vi "Found Four Edge.vi"(7 "Row ROI Name":string, 8 "error in":errorcluster, 9 "Calibration":T2, 10 "Template":T2, 11 "Image In":T2) -> (0 "error out":errorcluster, 1 "Array of Fitting":T1(array[cluster]), 2 "Match?":bool, 3 "Image out":T2, 4 "Elapsed time(ms)":u32)   [LabVIEW 2017]
uses:
  <vilib>/vision/Image Controls.llb/IMAQ Image.ctl
  Toolbox/Control/CVT Action.ctl
  <vilib>/vision/Measure.llb/Edge Options.ctl
  <vilib>/vision/Measure.llb/Edge Polarity.ctl
  <vilib>/vision/Measure.llb/Straight Edge Options.ctl
  <vilib>/vision/Measure.llb/Straight Edge Process.ctl
  Toolbox/Control/CVT name.vi
  Toolbox/Toolbox.lvlib
  <vilib>/vision/NI_Vision_Development_Module.lvlib
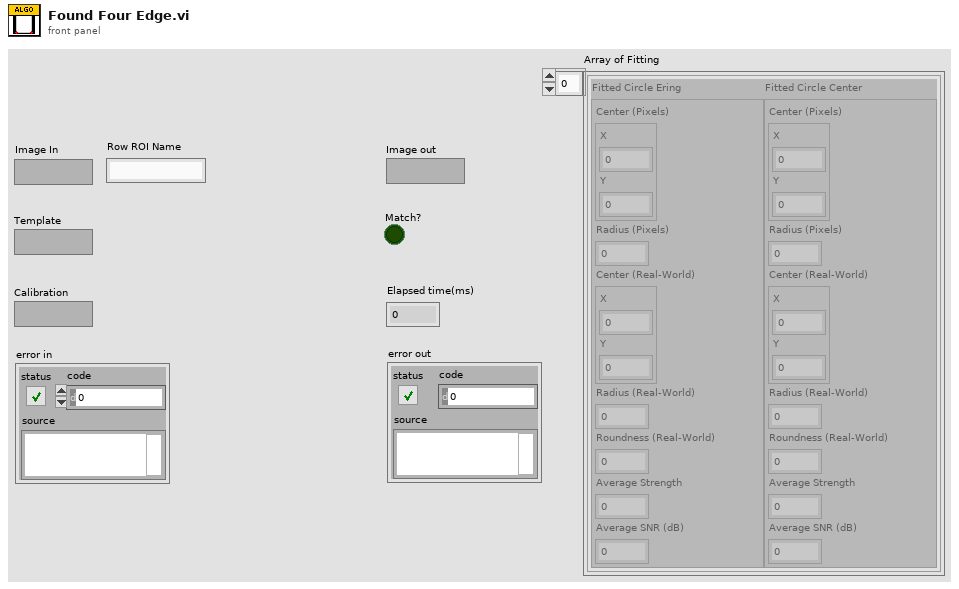
[diagram p1: front panel]
types:
  T1 = cluster{"Fitted Circle Ering":cluster{"Center (Pixels)":cluster{"X":sgl, "Y":sgl}, "Radius (Pixels)":dbl, "Center (Real-World)":cluster{"X":sgl, "Y":sgl}, "Radius (Real-World)":dbl, "Roundness (Real-World)":dbl, "Average Strength":dbl, "Average SNR (dB)":dbl}, "Fitted Circle Center":cluster{"Center (Pixels)":cluster{"X":sgl, "Y":sgl}, "Radius (Pixels)":dbl, "Center (Real-World)":cluster{"X":sgl, "Y":sgl}, "Radius (Real-World)":dbl, "Roundness (Real-World)":dbl, "Average Strength":dbl, "Average SNR (dB)":dbl}}[]
  T2 = typedef "IMAQ Image.ctl" = refnum<image>
  T3 = cluster{"State":string, "Image":T2, "Template":T2, "Calibration":T2, "Matches (pixel)":cluster{"Position":cluster{"x":sgl, "y":sgl}, "Angle":sgl, "Scale":sgl, "Score":sgl, "Bounding Box":cluster{"x":sgl, "y":sgl}[]}[], "Angle":dbl[], "Match?":bool, "start time(ms)":u32, "Array of Fitting":cluster{"Fitted Circle Ering":cluster{"Center (Pixels)":cluster{"X":sgl, "Y":sgl}, "Radius (Pixels)":dbl, "Center (Real-World)":cluster{"X":sgl, "Y":sgl}, "Radius (Real-World)":dbl, "Roundness (Real-World)":dbl, "Average Strength":dbl, "Average SNR (dB)":dbl}, "Fitted Circle Center":cluster{"Center (Pixels)":cluster{"X":sgl, "Y":sgl}, "Radius (Pixels)":dbl, "Center (Real-World)":cluster{"X":sgl, "Y":sgl}, "Radius (Real-World)":dbl, "Roundness (Real-World)":dbl, "Average Strength":dbl, "Average SNR (dB)":dbl}}[], "Row ROI Name":string}
  T4 = cluster{"Algorithm":i32, "Parameters":cluster{"Number of Matches Requested":i32, "Minimum Match Score":sgl, "Angle Ranges":cluster{"Start Angle":sgl, "End Angle":sgl}[]}, "Advanced Options":cluster{"Item":u16, "Value":dbl}[]}
  T5 = cluster{"Show Search Area":bool, "Show Features":bool, "Show Result":bool, "Show Label":bool, "Show Center":bool}
  T6 = typedef "Toolbox.lvlib/CVT Action.ctl" = enum16{"Set", "Replace", "Get", "Check", "Delete", "Delete All"}
  T7 = typedef "ROI Descriptor" = cluster{"Global Rectangle":i32[], "Contours":cluster{"ID":enum32{"External", "Internal"}, "Type":u32, "Coordinates":i32[]}[]}
  T8 = typedef "Edge Options.ctl" = cluster{"Edge Polarity":T9, "Kernel Size":u32, "Width":u32, "Minimum Edge Strength":sgl, "Interpolation Type":enum32{"Zero Order", "Bilinear", "Quadratic", "Cubic", "Bilinear Fixed"}, "Data Processing Method":enum32{"Average", "Median"}}
  T9 = typedef "Edge Polarity.ctl" = u32
  T10 = cluster{"Options":cluster{"Search  Direction":u32, "Edge Options":T8, "Show Search Area":bool, "Show Search Lines":bool, "Show Edges Found":bool, "Show Result":bool, "Search Area Color":u32, "Search Lines Color":u32, "Edge Locations Color":u32, "Result Color":u32, "Overlay Group Name":string}, "Circle Fit Options":cluster{"Process":enum16{"Get First Edge", "Get First + Last Edge", "Get All Edges", "Get Best Edge"}, "Step Size":dbl, "Max Pixel Radius":i32}}
  T11 = typedef "Straight Edge Options.ctl" = cluster{"Number of Lines":i32, "Type":T12, "Min. Score":dbl, "Max. Score":dbl, "Orientation":dbl, "Angle Range":dbl, "Angle Tolerance":dbl, "Step Size":u32, "Min. SNR (db)":dbl, "Min. Points (%)":dbl, "Hough Iterations":i32}
  T12 = typedef "Straight Edge Process.ctl" = enum32{"First Edge Rake", "Best Edge Rake", "Hough Edge Rake", "First Edge Projection", "Best Edge Projection"}
  T13 = cluster{"Options":cluster{"Search Direction":u32, "Edge Options":T8, "Show Search Area":bool, "Show Search Lines":bool, "Show Edges Found":bool, "Show Result":bool, "Search Area Color":u32, "Search Lines Color":u32, "Edge Locations Color":u32, "Result Color":u32, "Overlay Group Name":string}, "Line Fit Options":T11}
  T14 = cluster{"Position":cluster{"x":sgl, "y":sgl}, "Angle":sgl, "Scale":sgl, "Score":sgl, "Bounding Box":cluster{"x":sgl, "y":sgl}[]}[]
  T15 = cluster{"Fitted Circle Ering":cluster{"Center (Pixels)":cluster{"X":sgl, "Y":sgl}, "Radius (Pixels)":dbl, "Center (Real-World)":cluster{"X":sgl, "Y":sgl}, "Radius (Real-World)":dbl, "Roundness (Real-World)":dbl, "Average Strength":dbl, "Average SNR (dB)":dbl}, "Fitted Circle Center":cluster{"Center (Pixels)":cluster{"X":sgl, "Y":sgl}, "Radius (Pixels)":dbl, "Center (Real-World)":cluster{"X":sgl, "Y":sgl}, "Radius (Real-World)":dbl, "Roundness (Real-World)":dbl, "Average Strength":dbl, "Average SNR (dB)":dbl}}
  T16 = cluster{"Position":cluster{"x":sgl, "y":sgl}, "Angle":sgl, "Scale":sgl, "Score":sgl, "Bounding Box":cluster{"x":sgl, "y":sgl}[]}
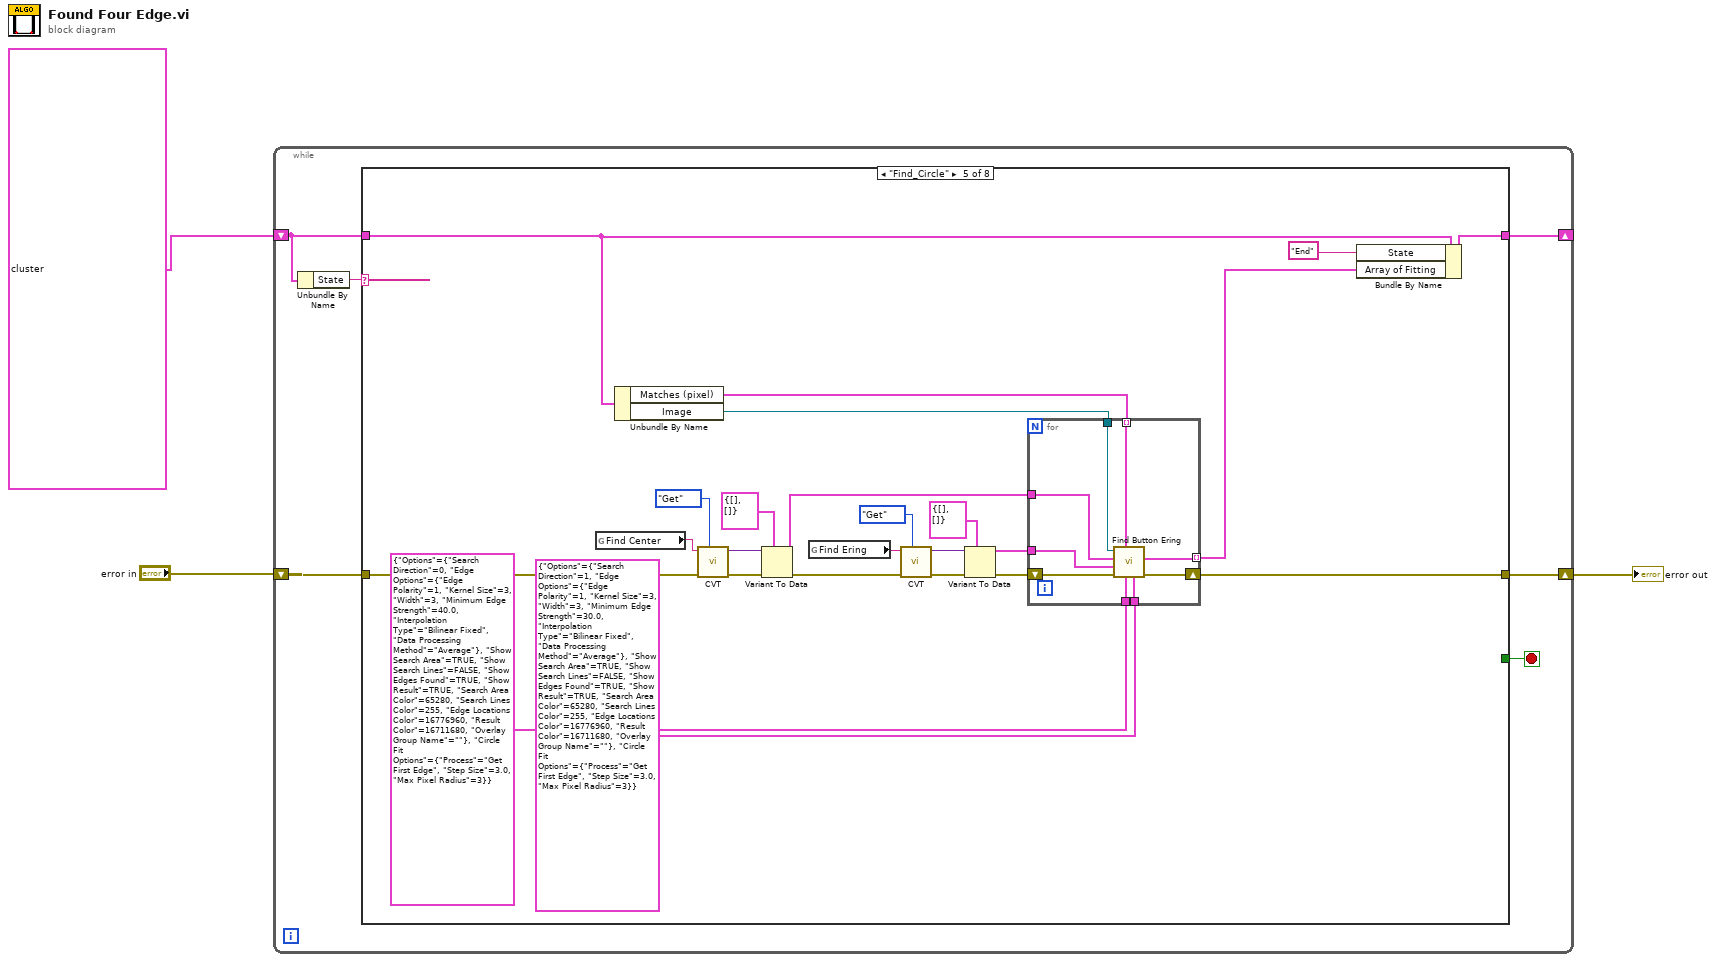
[diagram p0: block diagram]
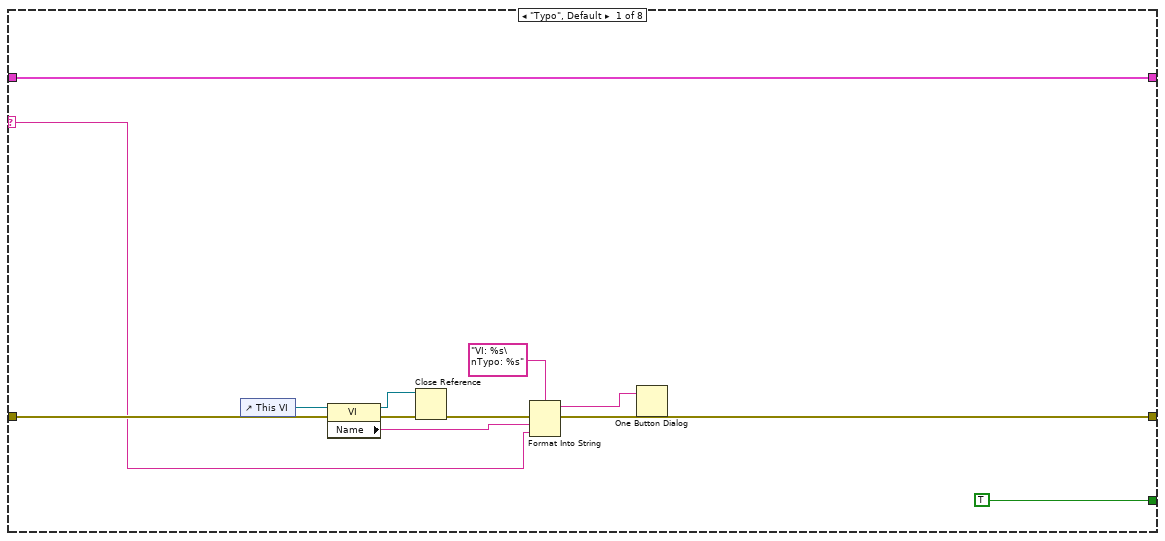
[diagram p2: hidden frame]
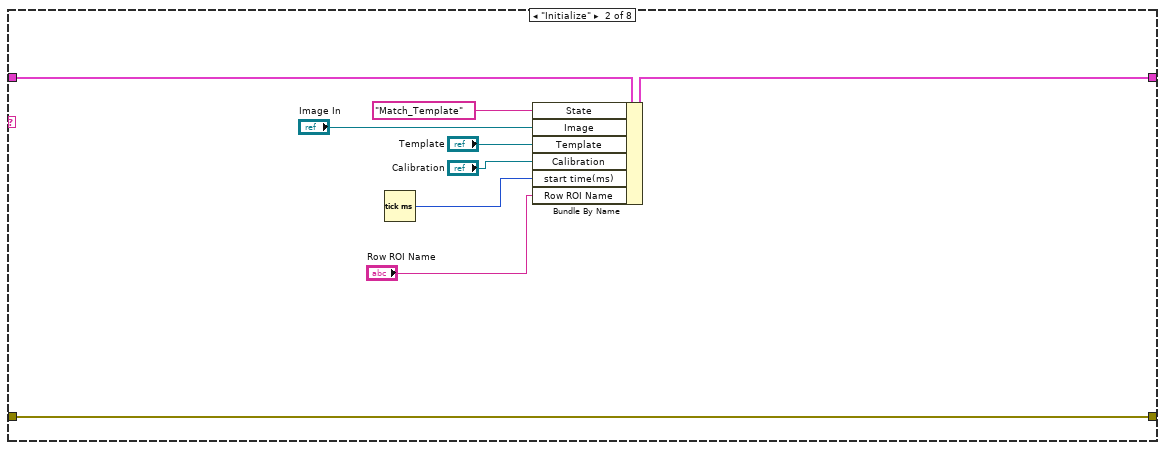
[diagram p3: hidden frame]
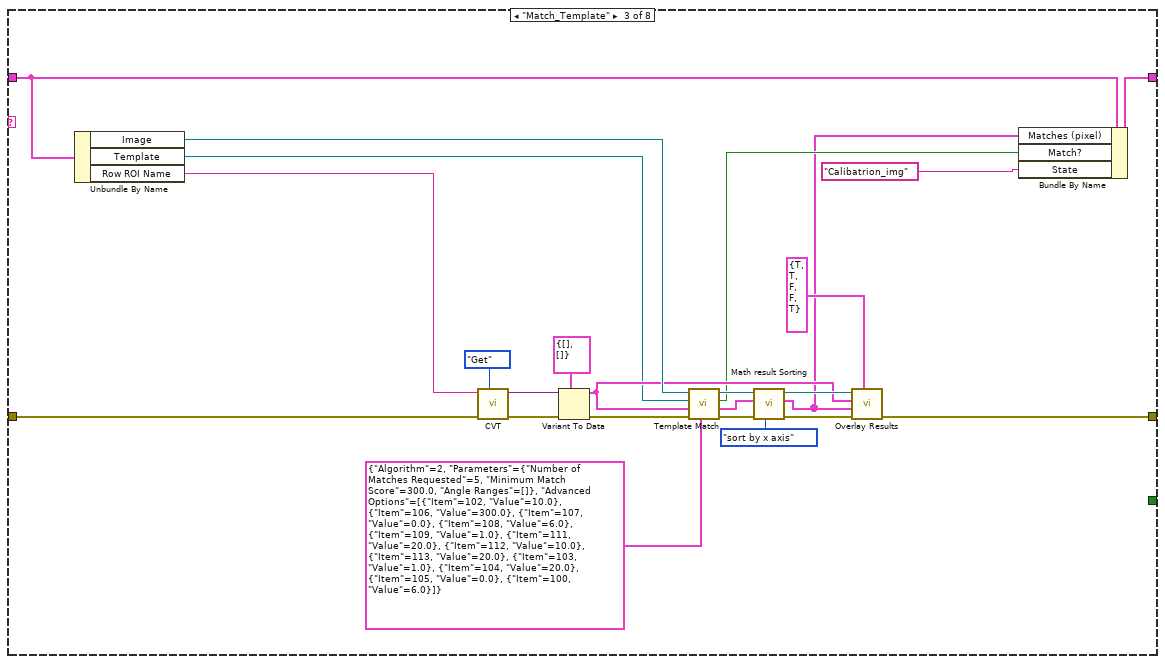
[diagram p4: hidden frame]
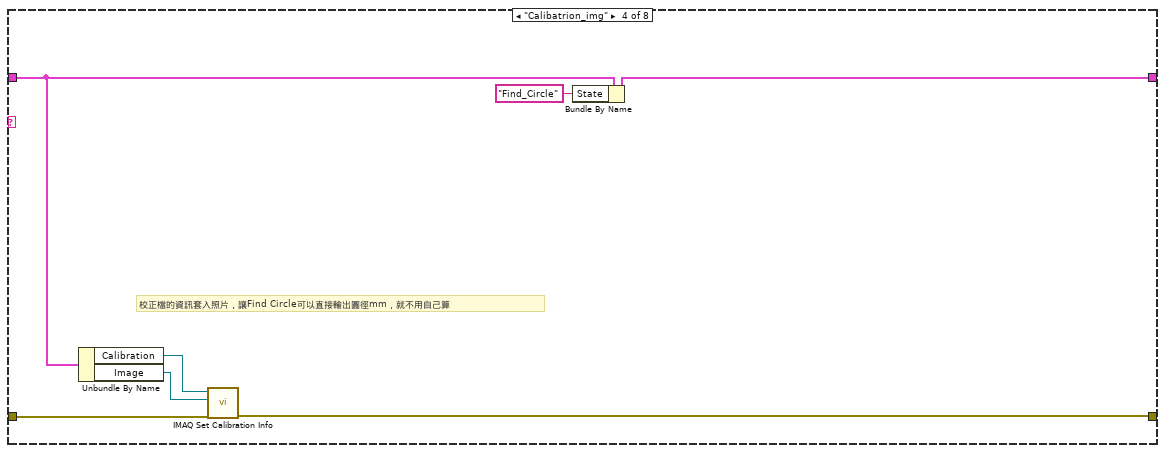
[diagram p5: hidden frame]
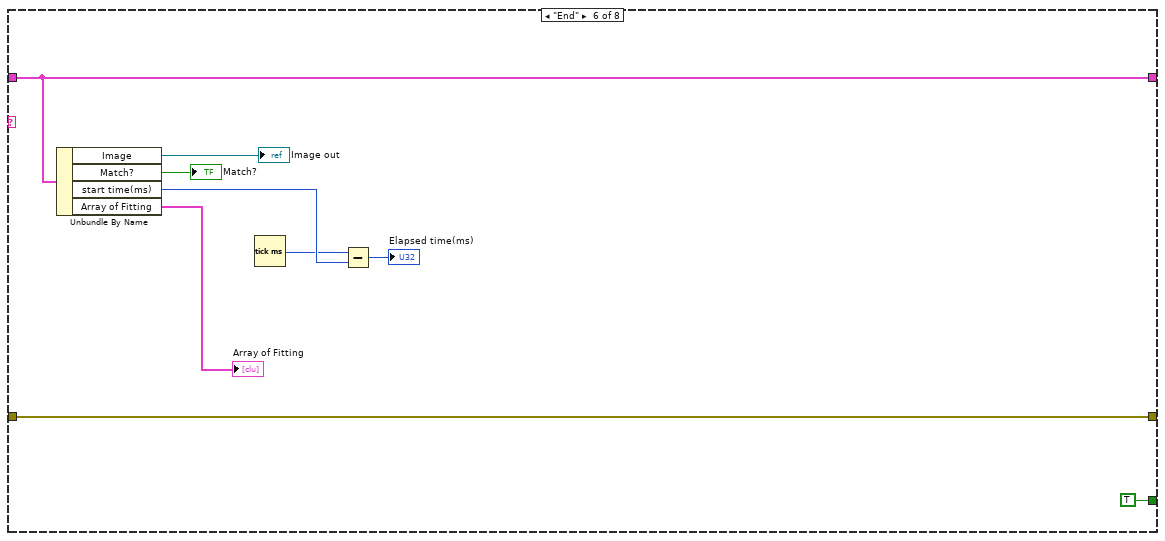
[diagram p6: hidden frame]
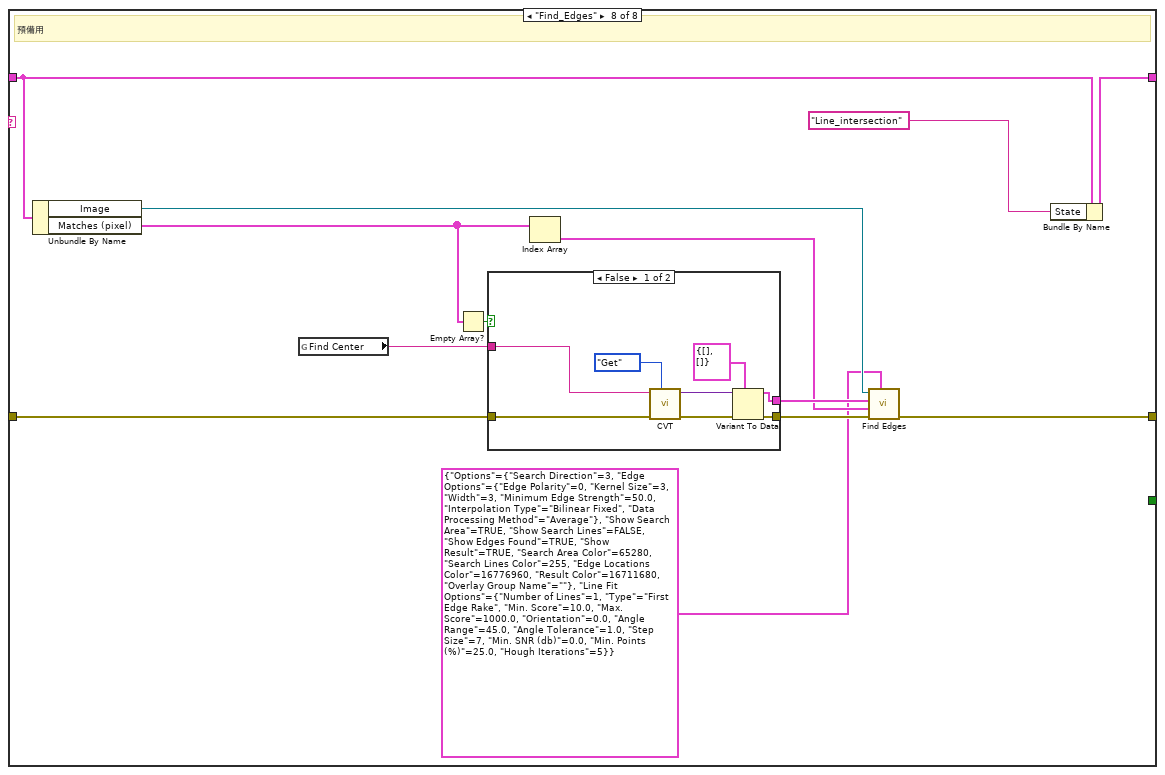
[diagram p8: hidden frame]
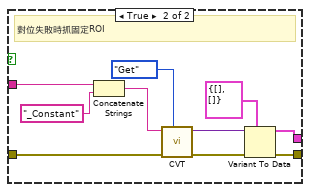
[diagram p9: hidden frame]
diagram:
  n1 = while {
    shift-right: [w9] -> _
    shift-left: T3 {"State"="Initialize", "Image"=refnum, "Template"=refnum, "Calibration"=refnum, "Matches (pixel)"=[], "Angle"=[], "Match?"=FALSE, "start time(ms)"=0, "Array of Fitting"=[], "Row ROI Name"=""} -> [w8]
    shift-right: [w6] -> w1
    shift-left: "error in" -> [w5]
    stop <- w4 stop-if-true
    n2 = Unbundle By Name(w8) -> ("State"=w7:string)
    n3 = case shown="\"Find_Circle\"" w7 {
      selector: w7 -> [w10 _ _ _ _ _ _ _]
      tunnel: [w21 w28 w50 w55 w83 w100 w104 w112] -> w9
      tunnel: w8 -> [w21 w30 w49 w58 w84 w100 w104 w115]
      tunnel: [w16 w29 w51 w59 w73 w102 w103 w116] -> w6
      tunnel: w5 -> [w18 w29 w52 w60 w82 w102 w103 w117]
      tunnel: [TRUE _ _ _ _ TRUE _ _] -> w4
      frame "Typo", Default {
        n4 = control-ref of="This VI"() -> (w20:refnum<vi>)
        n5 = property class="VI"(reference=w20, error in=w18) -> (reference out=w14:refnum<vi>, error out=w17:errorcluster, "Name"=w11:string)
        n6 = Close Reference(reference=w14, error in (no error)=w17) -> (error out=w15:errorcluster)
        n7 = Format Into String(format string="VI: %s\nTypo: %s", error in=w15, w11, w10) -> (resulting string=w12:string, error out=w16:errorcluster)  [unwired: 1 in]
        n8 = One Button Dialog(message=w12) -> ()  [unwired: 1 in, 1 out]
      }
      frame "Initialize" {
        n9 = Tick Count (ms)() -> (millisecond timer value=w24:u32)
        n10 = Bundle By Name(cluster=w30, "State"="Match_Template", "Image"="Image In", "Template"="Template", "Calibration"="Calibration", "start time(ms)"=w24, "Row ROI Name"="Row ROI Name") -> (w28:T3)
      }
      frame "Match_Template" {
        n11 = Unbundle By Name(w49) -> ("Image"=w48:T2, "Template"=w40:T2, "Row ROI Name"=w36:string)
        n12 = call "CVT.vi"("Action"=CVT_Action."Get", "error in (no error)"=w52, "Key"=w36) -> ("error out"=w47:errorcluster, "Value out"=w45:variant)  [unwired: 6 in, 1 out]
        n13 = Variant To Data(error in=w47, type=T7 {"Global Rectangle"=[], "Contours"=[]} ("ROI Descriptor"), Variant=w45) -> (data=w41:T7, error out=w46:errorcluster)
        n14 = call "Template Match.vi"("Match setup"=T4 {"Algorithm"=2, "Parameters"={"Number of Matches Requested"=5, "Minimum Match Score"=300.0, "Angle Ranges"=[]}, "Advanced Options"=[{"Item"=102, "Value"=10.0}, {"Item"=106, "Value"=300.0}, {"Item"=107, "Value"=0.0}, {"Item"=108, "Value"=6.0}, {"Item"=109, "Value"=1.0}, {"Item"=111, "Value"=20.0}, {"Item"=112, "Value"=10.0}, {"Item"=113, "Value"=20.0}, {"Item"=103, "Value"=1.0}, {"Item"=104, "Value"=20.0}, {"Item"=105, "Value"=0.0}, {"Item"=100, "Value"=6.0}]}, "error in (no error)"=w46, "ROI Descriptor"=w41, "Template Image"=w40, "Image In"=w48) -> ("error out"=w35:errorcluster, "Matches (pixel)"=w33:T14, "Match?"=w38:bool, "Image Out"=w53:T2)  [unwired: 3 in]
        n15 = call "Math result Sorting.vi"("sort method"=enum16{"sort by x axis", "sort by y axis"}."sort by x axis", "error in"=w35, "Matches (pixel)"=w33) -> ("error out"=w34:errorcluster, "Matches (pixel)"=w32:T14)  [unwired: 7 in]
        n16 = call "Overlay Results.vi"("Overlay Setup"=T5 {"Show Search Area"=TRUE, "Show Features"=TRUE, "Show Result"=FALSE, "Show Label"=FALSE, "Show Center"=TRUE}, "error in (no error)"=w34, "Matches (pixels)"=w32, "Search Area"=w41, "Image In"=w53) -> ("error out"=w51:errorcluster)  [unwired: 4 in, 2 out]
        n17 = Bundle By Name(cluster=w49, "Matches (pixel)"=w32, "Match?"=w38, "State"="Calibatrion_img") -> (w50:T3)
      }
      frame "Calibatrion_img" {
        # "校正檔的資訊套入照片，讓Find Circle可以直接輸出圓徑mm，就不用自己算"
        n18 = Unbundle By Name(w58) -> ("Calibration"=w57:T2, "Image"=w56:T2)
        n19 = call "IMAQ Set Calibration Info"("error in (no error)"=w60, "Image Dst"=w56, "Image Src"=w57) -> ("error out"=w59:errorcluster)  [unwired: 7 in, 1 out]
        n20 = Bundle By Name(cluster=w58, "State"="Find_Circle") -> (w55:T3)
      }
      frame "Find_Circle" {
        n21 = global read "CVT name.vi" "Find Center"() -> (w79:string)
        n22 = Unbundle By Name(w84) -> ("Matches (pixel)"=w62:T14, "Image"=w74:T2)
        n23 = call "CVT.vi"("Action"=CVT_Action."Get", "error in (no error)"=w82, "Key"=w79) -> ("error out"=w81:errorcluster, "Value out"=w76:variant)  [unwired: 6 in, 1 out]
        n24 = Variant To Data(error in=w81, type=T7 {"Global Rectangle"=[], "Contours"=[]} ("ROI Descriptor"), Variant=w76) -> (data=w75:T7, error out=w65:errorcluster)
        n25 = global read "CVT name.vi" "Find Ering"() -> (w69:string)
        n26 = call "CVT.vi"("Action"=CVT_Action."Get", "error in (no error)"=w65, "Key"=w69) -> ("error out"=w68:errorcluster, "Value out"=w70:variant)  [unwired: 6 in, 1 out]
        n27 = Variant To Data(error in=w68, type=T7 {"Global Rectangle"=[], "Contours"=[]} ("ROI Descriptor"), Variant=w70) -> (data=w63:T7, error out=w64:errorcluster)
        n28 = for {
          tunnel: T10 {"Options"={"Search  Direction"=0, "Edge Options"={"Edge Polarity"=1, "Kernel Size"=3, "Width"=3, "Minimum Edge Strength"=40.0, "Interpolation Type"=enum."Bilinear Fixed", "Data Processing Method"=enum."Average"}, "Show Search Area"=TRUE, "Show Search Lines"=FALSE, "Show Edges Found"=TRUE, "Show Result"=TRUE, "Search Area Color"=65280, "Search Lines Color"=255, "Edge Locations Color"=16776960, "Result Color"=16711680, "Overlay Group Name"=""}, "Circle Fit Options"={"Process"=enum."Get First Edge", "Step Size"=3.0, "Max Pixel Radius"=3}} ("Find Circle Setting") -> [w89]
          tunnel: w75 -> [w86]
          tunnel: w74 -> [w93]
          tunnel: T10 {"Options"={"Search  Direction"=1, "Edge Options"={"Edge Polarity"=1, "Kernel Size"=3, "Width"=3, "Minimum Edge Strength"=30.0, "Interpolation Type"=enum."Bilinear Fixed", "Data Processing Method"=enum."Average"}, "Show Search Area"=TRUE, "Show Search Lines"=FALSE, "Show Edges Found"=TRUE, "Show Result"=TRUE, "Search Area Color"=65280, "Search Lines Color"=255, "Edge Locations Color"=16776960, "Result Color"=16711680, "Overlay Group Name"=""}, "Circle Fit Options"={"Process"=enum."Get First Edge", "Step Size"=3.0, "Max Pixel Radius"=3}} ("Find Circle Setting") -> [w88]
          tunnel: w62 -> [w92] mode=indexing
          shift-right: [w90] -> w73
          shift-left: w64 -> [w91]
          tunnel: w63 -> [w87]
          tunnel: [w85] -> w61 mode=indexing
          n29 = call "Find Button Ering.vi"("Find Ering Setting"=w88, "Find Center Setting"=w89, "Match Position"=w92, "error in (no error)"=w91, "Ering ROI"=w87, "Center ROI"=w86, "Image in"=w93) -> ("error out"=w90:errorcluster, "Array of Fittings"=w85:T15)  [unwired: 3 in]
        }
        n30 = Bundle By Name(cluster=w84, "State"="End", "Array of Fitting"=w61) -> (w83:T3)
      }
      frame "End" {
        n31 = Unbundle By Name(w100) -> ("Image"=→"Image out":T2, "Match?"=→"Match?":bool, "start time(ms)"=w97:u32, "Array of Fitting"=→"Array of Fitting":T1)
        n32 = Tick Count (ms)() -> (millisecond timer value=w96:u32)
        n33 = Subtract(x=w96, y=w97) -> (x-y=→"Elapsed time(ms)":u32)
      }
      frame "--old backup--" {
      }
      frame "Find_Edges" {
        # "預備用"
        n34 = Unbundle By Name(w115) -> ("Image"=w113:T2, "Matches (pixel)"=w114:T14)
        n35 = global read "CVT name.vi" "Find Center"() -> (w105:string)
        n36 = Empty Array?(array=w114) -> (empty?=w107:bool)
        n37 = case shown="False" w107 {
          tunnel: w117 -> [w121 w132]
          tunnel: w105 -> [w118 w130]
          tunnel: [w120 w129] -> w110
          tunnel: [w119 w128] -> w109
          frame False {
            n38 = call "CVT.vi"("Action"=CVT_Action."Get", "error in (no error)"=w121, "Key"=w118) -> ("error out"=w124:errorcluster, "Value out"=w125:variant)  [unwired: 6 in, 1 out]
            n39 = Variant To Data(error in=w124, type=T7 {"Global Rectangle"=[], "Contours"=[]} ("ROI Descriptor"), Variant=w125) -> (data=w119:T7, error out=w120:errorcluster)
          }
          frame True {
            # "對位失敗時抓固定ROI"
            n40 = Concatenate Strings(w130, "_Constant" ("string")) -> (w127:string)
            n41 = call "CVT.vi"("Action"=CVT_Action."Get", "error in (no error)"=w132, "Key"=w127) -> ("error out"=w134:errorcluster, "Value out"=w135:variant)  [unwired: 6 in, 1 out]
            n42 = Variant To Data(error in=w134, type=T7 {"Global Rectangle"=[], "Contours"=[]} ("ROI Descriptor"), Variant=w135) -> (data=w128:T7, error out=w129:errorcluster)
          }
        }
        n43 = Index Array(array=w114) -> (element=w108:T16)  [unwired: 1 in]
        n44 = call "Find Edges.vi"("Find Edge setting"=T13 {"Options"={"Search Direction"=3, "Edge Options"={"Edge Polarity"=0, "Kernel Size"=3, "Width"=3, "Minimum Edge Strength"=50.0, "Interpolation Type"=enum."Bilinear Fixed", "Data Processing Method"=enum."Average"}, "Show Search Area"=TRUE, "Show Search Lines"=FALSE, "Show Edges Found"=TRUE, "Show Result"=TRUE, "Search Area Color"=65280, "Search Lines Color"=255, "Edge Locations Color"=16776960, "Result Color"=16711680, "Overlay Group Name"=""}, "Line Fit Options"={"Number of Lines"=1, "Type"=enum."First Edge Rake", "Min. Score"=10.0, "Max. Score"=1000.0, "Orientation"=0.0, "Angle Range"=45.0, "Angle Tolerance"=1.0, "Step Size"=7, "Min. SNR (db)"=0.0, "Min. Points (%)"=25.0, "Hough Iterations"=5}}, "error in (no error)"=w110, "Matches (pixel)"=w108, "ROI Descriptor"=w109, "Image"=w113) -> ("error out"=w116:errorcluster)  [unwired: 3 in, 3 out]
        n45 = Bundle By Name(cluster=w115, "State"="Line_intersection") -> (w112:T3)
      }
    }
  }
  "error out" <- w1
